vi "PCB quality(TCP2Foxconn).vi"(7 "Bypass查詢":bool, 8 "error in (no error)":errorcluster, 10 "Barcode":string, 11 "TCP2Foxc":string="Driver={ODBC Driver 17 for SQL Server};Server=localhost\\SQLEXPRESS;Database=YDXB01;UID=labview;PWD=123456789") -> (0 "error out":errorcluster={"status"=TRUE, "code"=-2147217900, "source"="NI_Database_API.lvlib:Conn Execute.vi->NI_Database_API.lvlib:DB Tools Select Data.vi->Select WebCam BBOX.vi<ERR>ADO Error: 0x80040E14\r\nException occured in Microsoft OLE DB Provider for ODBC Drivers: [Microsoft][ODBC Driver 17 for SQL Server][SQL Server]接近 ',' 之處的語法不正確。 in NI_Database_API.lvlib:Conn Execute.vi->NI_Database_API.lvlib:DB Tools Select Data.vi->Select WebCam BBOX.vi"}, 2 "result":string)   [LabVIEW 2019, in "TCP2Foxconn.lvlib"]
uses:
  TCP2Foxconn.lvlib
panel:
  out "break":bool
  out "Connect?":bool
  out "times":i32
  # "True為OK"
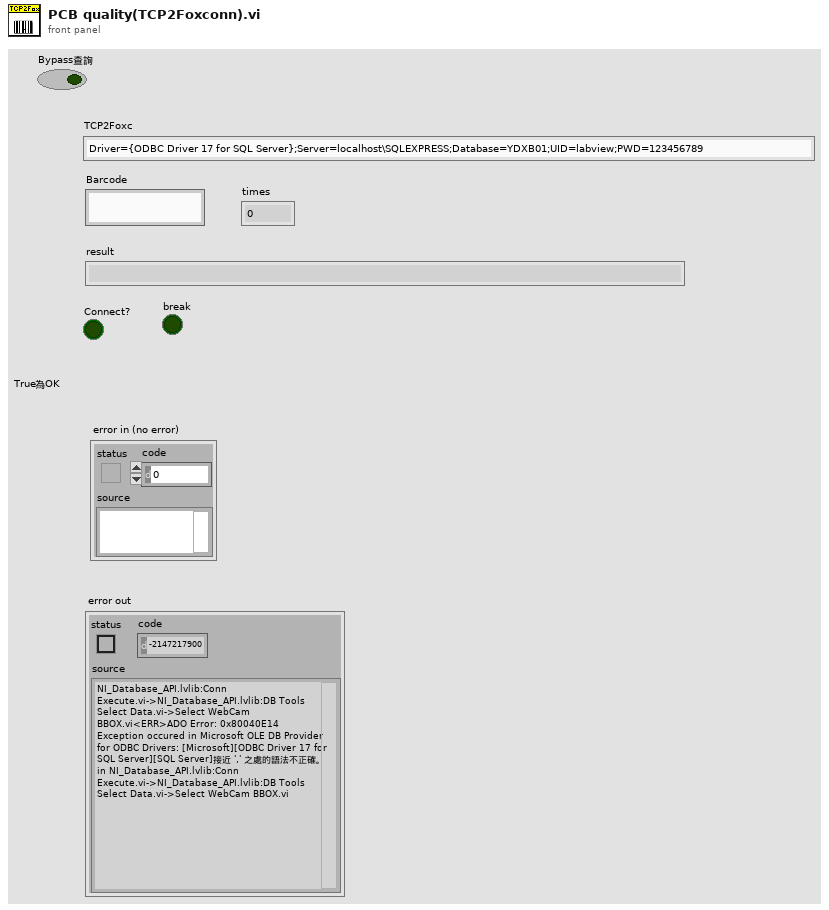
[diagram p1: front panel]
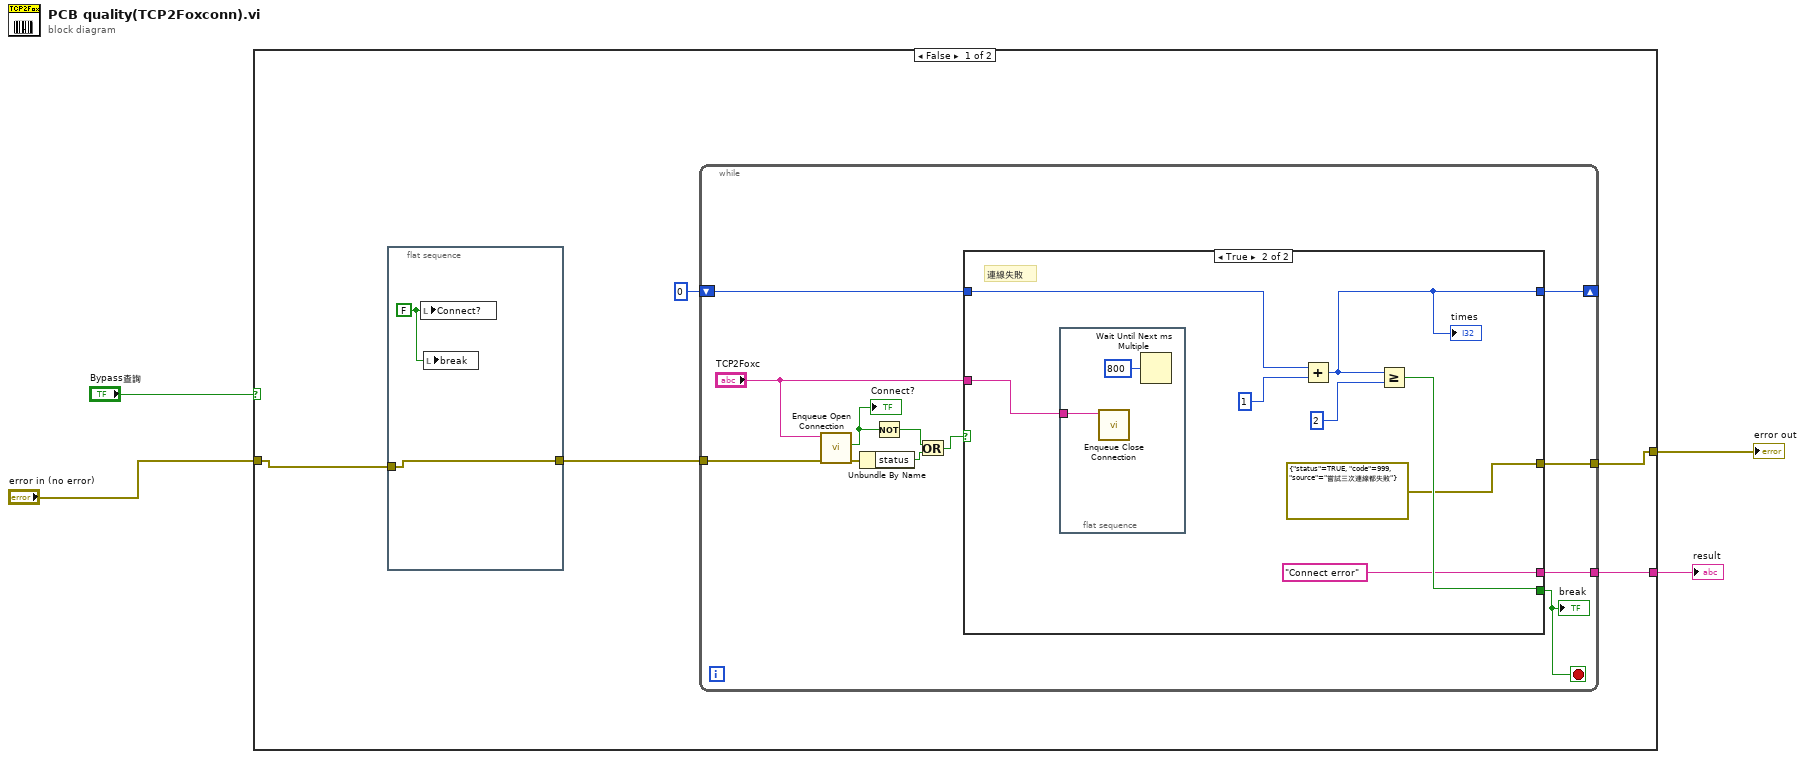
[diagram p0: block diagram]
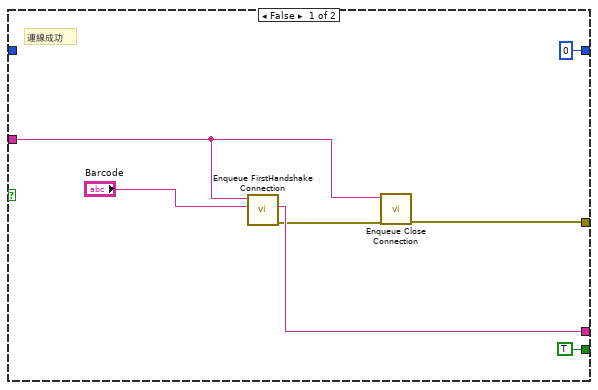
[diagram p2: hidden frame]
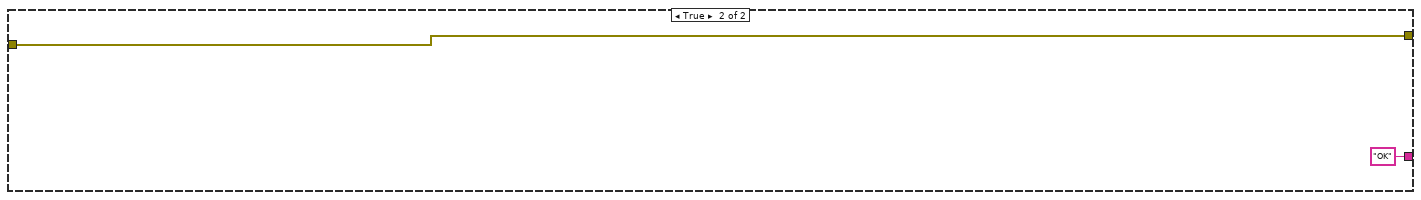
[diagram p3: hidden frame]
diagram:
  n1 = case shown="False" "Bypass查詢" {
    tunnel: [w9 "OK"] -> w4
    tunnel: "error in (no error)" -> [w6 w41]
    tunnel: [w8 w41] -> w1
    frame False {
      n2 = flat-sequence {
        tunnel: w6 -> [w10]
        tunnel: [w10] -> w5
        frame #0 {
          w11 = FALSE ("Connect?")
          n3 = local write "Connect?"(w11) -> ()
          n4 = local write "break"(w11) -> ()
        }
      }
      n5 = while {
        tunnel: w5 -> [w23]
        tunnel: [w16] -> w9
        tunnel: [w15] -> w8
        shift-right: [w13] -> _
        shift-left: 0 -> [w14]
        stop <- w12 stop-if-true
        n6 = call "Enqueue Open Connection.vi"("Error In"=w23, "Name"="TCP2Foxc") -> ("Error Out"=w22:errorcluster, "Connect?"=w21:bool)  [unwired: 8 in]
        "Connect?" <- w21
        n7 = Unbundle By Name(w22) -> ("status"=w20:bool)
        n8 = Not(x=w21) -> (.not. x?=w19:bool)
        n9 = Or(x=w19, y=w20) -> (x .or. y?=w18:bool)
        n10 = case shown="True" w18 {
          tunnel: "TCP2Foxc" -> [w26 w32]
          tunnel: [w29 "Connect error" ("Result")] -> w16
          tunnel: [w27 errorcluster {"status"=TRUE, "code"=999, "source"="嘗試三次連線都失敗"} ("error constant")] -> w15
          tunnel: w14 -> [_ w38]
          tunnel: [TRUE w35] -> w12
          tunnel: [0 w31] -> w13
          frame False {
            # "連線成功"
            n11 = call "Enqueue FirstHandshake Connection.vi"("Barcode"="Barcode", "Name"=w26) -> ("Error Out"=w28:errorcluster, "Result"=w29:string)  [unwired: 8 in]
            n12 = call "Enqueue Close Connection.vi"("Error In"=w28, "Name"=w26) -> ("Error Out"=w27:errorcluster)  [unwired: 9 in]
          }
          frame True {
            # "連線失敗"
            n13 = flat-sequence {
              tunnel: w32 -> [w39]
              frame #0 {
                n14 = call "Enqueue Close Connection.vi"("Name"=w39) -> ()  [unwired: 10 in, 1 out]
                n15 = Wait Until Next ms Multiple(millisecond multiple=u32 800) -> ()  [unwired: 1 out]
              }
            }
            n16 = Add(x=w38, y=1) -> (x+y=w31:i32)
            "times" <- w31
            n17 = Greater Or Equal?(x=w31, y=2) -> (x >= y?=w35:bool)
          }
        }
        "break" <- w12
      }
    }
    frame True {
    }
  }
  "result" <- w4
  "error out" <- w1
